vi "upload.vi"(7 "LabVIEW Web Service Request":refnum<class "Web Request.lvclass">) -> ()   [LabVIEW 2015]
uses:
  <vilib>/wsapi/Web Request.lvclass
  global_cms.vi
panel:
  # "Use the Web Service Request input terminal to call the VIs on the Web Services palette. Do not remove it from the connector pane unless you don't need access to the palette."
  # "Each additional control wired to the connector pane will be available as an input in the URL. To include an indicator in terminal-mode output (the default setting), it must also be wired to the connector pane."
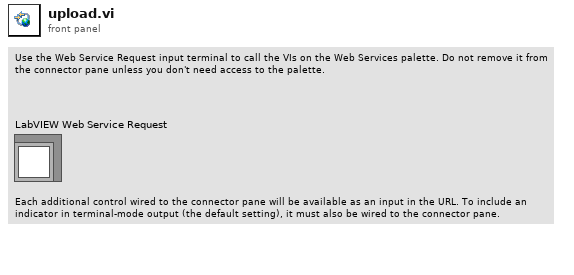
[diagram p1: front panel]
types:
  T1 = cluster{"data":cluster{"fileRequest":cluster{"filePath":string, "fileType":string, "fileName":string, "time":u32, "filePathTmp":string, "fileSize":u32}, "fileResponse":cluster{"filePath":string, "fileType":string, "fileName":string, "decode":string, "result":string, "status":string, "time":u32, "size":u32}}[], "_status":string, "_token":string}
  T2 = cluster{"fileRequest":cluster{"filePath":string, "fileType":string, "fileName":string, "time":u32, "filePathTmp":string, "fileSize":u32}, "fileReponse":cluster{"filePath":string, "fileType":string, "fileName":string, "decode":string, "result":string, "status":string, "time":u32, "size":u32}}
  T3 = cluster{"Local File Path":string, "Client File Name":string, "Content Type":string, "Size":u32}[]
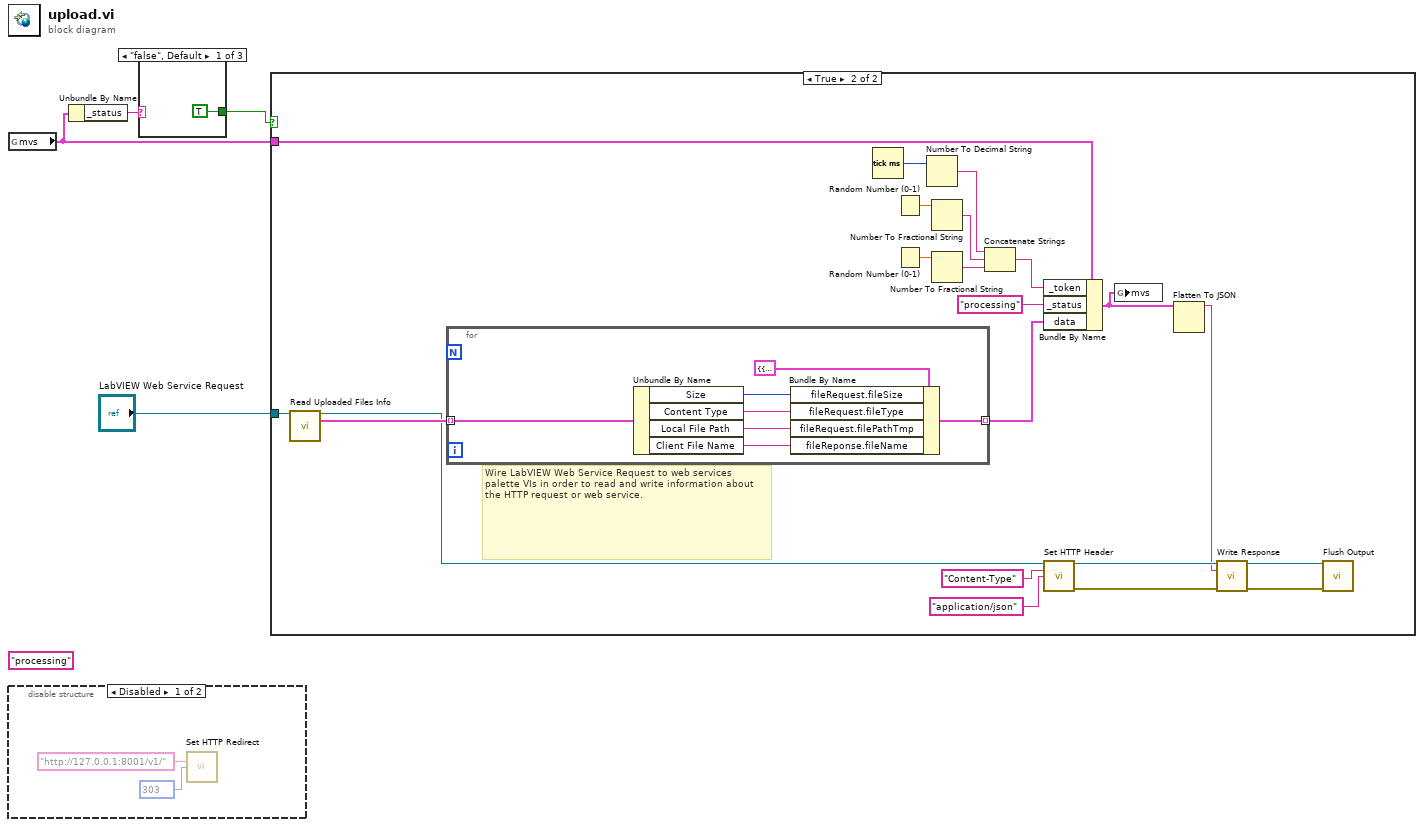
[diagram p0: block diagram]
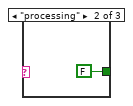
[diagram p2: hidden frame]
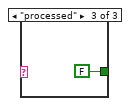
[diagram p3: hidden frame]
diagram:
  (unwired) "processing" ("_status")
  n1 = global read "global_cms.vi" "mvs"() -> (w3:T1)
  n2 = disable-structure shown="Disabled" {
    frame Disabled {
      w6 = 303 items=["100"=100, "101"=101, "200"=200, "201"=201, "202"=202, "203"=203, "204"=204, "205"=205, "206"=206, "300"=300, "301"=301, "302"=302, "303"=303, "304"=304, "305"=305, "306"=306, "307"=307, "400"=400, "401"=401, "402"=402, "403"=403, "404"=404, "405"=405, "406"=406, "407"=407, "408"=408, "409"=409, "410"=410, "411"=411, "412"=412, "413"=413, "414"=414, "415"=415, "416"=416, "417"=417, "500"=500, "501"=501, "502"=502, "503"=503, "504"=504, "505"=505] ("response code (307)")
      n3 = call <vilib>:"Set HTTP Redirect.vi"("redirect URL"="http://127.0.0.1:8001/v1/", "response code (307)"=w6) -> ()  [unwired: 12 in, 2 out]
    }
    frame Enabled {
    }
  }
  n4 = Unbundle By Name(w3) -> ("_status"=w2:string)
  n5 = case shown="\"false\", Default" w2 {
    tunnel: [TRUE FALSE FALSE] -> w1
    frame "false", Default {
    }
    frame "processing" {
    }
    frame "processed" {
    }
  }
  n6 = case shown="True" w1 {
    tunnel: "LabVIEW Web Service Request" -> [_ w30]
    tunnel: w3 -> [_ w19]
    frame False {
    }
    frame True {
      # "Wire LabVIEW Web Service Request to web services palette VIs in order to read and write information about the HTTP request or web service."
      n7 = call <vilib>:"Read Uploaded Files Info.vi"("LabVIEW Web Service Request"=w30) -> ("LabVIEW Web Service Request out"=w28:refnum<class "Web Request.lvclass">, "UploadedFilesList"=w29:T3)  [unwired: 12 in, 1 out]
      n8 = for {
        tunnel: w29 -> [w37] mode=indexing
        tunnel: [w31] -> w17 mode=indexing
        n9 = Unbundle By Name(w37) -> ("Size"=w33:u32, "Content Type"=w34:string, "Local File Path"=w35:string, "Client File Name"=w36:string)
        n10 = Bundle By Name(cluster=T2 {"fileRequest"={"filePath"="", "fileType"="", "fileName"="", "time"=0, "filePathTmp"="", "fileSize"=0}, "fileReponse"={"filePath"="", "fileType"="", "fileName"="", "decode"="", "result"="", "status"="", "time"=0, "size"=0}} ("fileData"), "fileRequest.fileSize"=w33, "fileRequest.fileType"=w34, "fileRequest.filePathTmp"=w35, "fileReponse.fileName"=w36) -> (w31:T2)
      }
      n11 = Tick Count (ms)() -> (millisecond timer value=w16:u32)
      n12 = Random Number (0-1)() -> (number: 0 to 1=w14:dbl)
      n13 = Random Number (0-1)() -> (number: 0 to 1=w12:dbl)
      n14 = Number To Decimal String(number=w16) -> (decimal integer string=w15:string)  [unwired: 1 in]
      n15 = Number To Fractional String(number=w14) -> (F-format string=w13:string)  [unwired: 3 in]
      n16 = Number To Fractional String(number=w12) -> (F-format string=w11:string)  [unwired: 3 in]
      n17 = Concatenate Strings(w15, w13, w11) -> (w10:string)
      n18 = Bundle By Name(cluster=w19, "_token"=w10, "_status"="processing", "data"=w17) -> (w18:T1)
      n19 = call <vilib>:"Set HTTP Header.vi"("LabVIEW Web Service Request"=w28, "header"="Content-Type", "header value"="application/json") -> ("LabVIEW Web Service Request out"=w23:refnum<class "Web Request.lvclass">, "error out"=w21:errorcluster)  [unwired: 11 in]
      n20 = global write "global_cms.vi" "mvs"(w18) -> ()
      n21 = Flatten To JSON(anything=w18) -> (JSON string=w22:string)  [unwired: 2 in, 1 out]
      n22 = call <vilib>:"Write Response.vi"("LabVIEW Web Service Request"=w23, "response string"=w22, "error in (no error)"=w21) -> ("LabVIEW Web Service Request out"=w25:refnum<class "Web Request.lvclass">, "error out"=w24:errorcluster)  [unwired: 11 in]
      n23 = call <vilib>:"Flush Output.vi"("LabVIEW Web Service Request"=w25, "error in (no error)"=w24) -> ()  [unwired: 12 in, 2 out]
    }
  }
